vi "hp3478a read.vi"(1 "HP 3478 ADDR":i16=3) -> (0 "Reading":dbl format="%.2e")   [LabVIEW 2015]
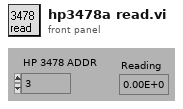
[diagram p1: front panel]
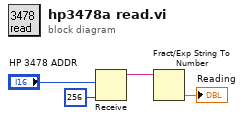
[diagram p0: block diagram]
diagram:
  n1 = Receive(6:256 ("count"), 8:"HP 3478 ADDR") -> (3:w4:string)  [unwired: 3 in, 3 out]
  n2 = Fract/Exp String To Number(string=w4) -> (number=→"Reading":dbl)  [unwired: 3 in, 1 out]
